vi "PathPlanner_Ctrl_HolonomicDrvExecute.vi"(6 "Period":dbl=0.02, 7 "PathPlanner_Ctrl_HolDrvConfig":T10={"HOLONOMIC_CTRL_PACK_TUNING"={"X PID Tuning"={"Kp"=0.0, "Ki"=0.0, "Kd"=0.0, "MaximumIntegral"=9.9e+30, "MinimumIntegral"=-9.9e+30}, "Y PID Tuning"={"Kp"=0.0, "Ki"=0.0, "Kd"=0.0, "MaximumIntegral"=9.9e+30, "MinimumIntegral"=-9.9e+30}, "thetaProfiledPID_CTRL"={"Controller"={"Kp"=0.0, "Ki"=0.0, "Kd"=0.0, "Period"=0.0, "Max_Integral"=1.0, "Min_Integral"=-1.0, "Max_Input"=0.0, "Min_Input"=0.0, "Continuous"=FALSE, "PositionError"=0.0, "VelocityError"=0.0, "PrevError"=0.0, "TotalError"=0.0, "PositionTolerance"=0.05, "VelocityTolerance"=9.99e+35, "SetPoint"=0.0, "Kf"=0.0, "Prev_Deriv"=0.0, "Prev_Deriv 2"=0.0, "DerivativeFilter"=FALSE, "Min_Output"=-9.99e+35, "Max_Output"=9.9e+35, "Prev_F_P"=0.0, "Prev_F_P_2"=0.0, "AntiWindupActive"=FALSE, "Measurement"=0.0}, "Goal"={"Position"=0.0, "Velocity"=0.0}, "Setpoint"={"Position"=0.0, "Velocity"=0.0}, "Constraint"={"MaxVelocity"=0.0, "MaxAcceleration"=0.0}}}, "Max Wheel Speed M/S"=0.0, "Tolerance SI"={"TRANSLATION"={"X"=0.04, "Y"=0.04}, "ROTATION"={"VALUE"=0.034906585039887, "COS"=0.999390827019096, "SIN"=0.034899496702501}}, "Drive Base Radius M"=0.0} {"Tolerance SI"."ROTATION"."SIN" format="%13.4f"; "Tolerance SI"."ROTATION"."COS" format="%13.4f"; "Tolerance SI"."ROTATION"."VALUE" format="%13.4f"; "Tolerance SI"."TRANSLATION"."Y" format="%14.3f"; "Tolerance SI"."TRANSLATION"."X" format="%14.3f"; "HOLONOMIC_CTRL_PACK_TUNING"."thetaProfiledPID_CTRL"."Constraint"."MaxAcceleration" format="%16_6e"; "HOLONOMIC_CTRL_PACK_TUNING"."thetaProfiledPID_CTRL"."Constraint"."MaxVelocity" format="%16_6e"; "HOLONOMIC_CTRL_PACK_TUNING"."thetaProfiledPID_CTRL"."Setpoint"."Velocity" format="%16_6e"; "HOLONOMIC_CTRL_PACK_TUNING"."thetaProfiledPID_CTRL"."Setpoint"."Position" format="%16_6e"; "HOLONOMIC_CTRL_PACK_TUNING"."thetaProfiledPID_CTRL"."Goal"."Velocity" format="%16_6e"; "HOLONOMIC_CTRL_PACK_TUNING"."thetaProfiledPID_CTRL"."Goal"."Position" format="%16_6e"; "HOLONOMIC_CTRL_PACK_TUNING"."thetaProfiledPID_CTRL"."Controller"."Measurement" format="%16_6e"; "HOLONOMIC_CTRL_PACK_TUNING"."thetaProfiledPID_CTRL"."Controller"."Prev_F_P_2" format="%16_6e"; "HOLONOMIC_CTRL_PACK_TUNING"."thetaProfiledPID_CTRL"."Controller"."Prev_F_P" format="%16_6e"; "HOLONOMIC_CTRL_PACK_TUNING"."thetaProfiledPID_CTRL"."Controller"."Max_Output" format="%16_6e"; "HOLONOMIC_CTRL_PACK_TUNING"."thetaProfiledPID_CTRL"."Controller"."Min_Output" format="%16_6e"; "HOLONOMIC_CTRL_PACK_TUNING"."thetaProfiledPID_CTRL"."Controller"."Prev_Deriv 2" format="%16_6e"; "HOLONOMIC_CTRL_PACK_TUNING"."thetaProfiledPID_CTRL"."Controller"."Prev_Deriv" format="%16_6e"; "HOLONOMIC_CTRL_PACK_TUNING"."thetaProfiledPID_CTRL"."Controller"."Kf" format="%16_6e"; "HOLONOMIC_CTRL_PACK_TUNING"."thetaProfiledPID_CTRL"."Controller"."SetPoint" format="%16_6e"; "HOLONOMIC_CTRL_PACK_TUNING"."thetaProfiledPID_CTRL"."Controller"."VelocityTolerance" format="%16_6e"; "HOLONOMIC_CTRL_PACK_TUNING"."thetaProfiledPID_CTRL"."Controller"."PositionTolerance" format="%16_6e"; "HOLONOMIC_CTRL_PACK_TUNING"."thetaProfiledPID_CTRL"."Controller"."TotalError" format="%16_6e"; "HOLONOMIC_CTRL_PACK_TUNING"."thetaProfiledPID_CTRL"."Controller"."PrevError" format="%16_6e"; "HOLONOMIC_CTRL_PACK_TUNING"."thetaProfiledPID_CTRL"."Controller"."VelocityError" format="%16_6e"; "HOLONOMIC_CTRL_PACK_TUNING"."thetaProfiledPID_CTRL"."Controller"."PositionError" format="%16_6e"; "HOLONOMIC_CTRL_PACK_TUNING"."thetaProfiledPID_CTRL"."Controller"."Min_Input" format="%16_6e"; "HOLONOMIC_CTRL_PACK_TUNING"."thetaProfiledPID_CTRL"."Controller"."Max_Input" format="%16_6e"; "HOLONOMIC_CTRL_PACK_TUNING"."thetaProfiledPID_CTRL"."Controller"."Min_Integral" format="%16_6e"; "HOLONOMIC_CTRL_PACK_TUNING"."thetaProfiledPID_CTRL"."Controller"."Max_Integral" format="%16_6e"; "HOLONOMIC_CTRL_PACK_TUNING"."thetaProfiledPID_CTRL"."Controller"."Period" format="%16_6e"; "HOLONOMIC_CTRL_PACK_TUNING"."thetaProfiledPID_CTRL"."Controller"."Kd" format="%16_6e"; "HOLONOMIC_CTRL_PACK_TUNING"."thetaProfiledPID_CTRL"."Controller"."Ki" format="%16_6e"; "HOLONOMIC_CTRL_PACK_TUNING"."thetaProfiledPID_CTRL"."Controller"."Kp" format="%16_6e"}, 8 "Enabled":bool=TRUE, 9 "Reset":bool, 10 "PathPlannerState":T13={"TimeSeconds"=0.0, "VelocityMPS"=0.0, "AccerationMpsSq"=0.0, "HeadingAngularVelRadPerSec"=0.0, "PositionMeters"={"X"=0.0, "Y"=0.0}, "Heading"={"VALUE"=0.0, "COS"=1.0, "SIN"=0.0}, "TargetHolonomicRotation"={"VALUE"=0.0, "COS"=1.0, "SIN"=0.0}, "CurvatureRadPerMeter"=0.0, "PathPlannerConstraints"={"MaxVelocityMps;"=0.0, "MaxAccelerationMpsSq;"=0.0, "MaxAngularVelRadPsEc;"=0.0, "MaxAngularAccRadPSecSq"=0.0, "Exists"=FALSE}, "DeltaPos"=0.0} {"TargetHolonomicRotation"."SIN" format="%13.4f"; "TargetHolonomicRotation"."COS" format="%13.4f"; "TargetHolonomicRotation"."VALUE" format="%13.4f"; "Heading"."SIN" format="%13.4f"; "Heading"."COS" format="%13.4f"; "Heading"."VALUE" format="%13.4f"; "PositionMeters"."Y" format="%14.3f"; "PositionMeters"."X" format="%14.3f"}, 11 "Current Pose SI":T3={"TRANSLATION"={"X"=0.0, "Y"=0.0}, "ROTATION"={"VALUE"=0.0, "COS"=1.0, "SIN"=0.0}} {"ROTATION"."SIN" format="%13.4f"; "ROTATION"."COS" format="%13.4f"; "ROTATION"."VALUE" format="%13.4f"; "TRANSLATION"."Y" format="%14.3f"; "TRANSLATION"."X" format="%14.3f"}) -> (1 "Position Error M":dbl, 2 "At Reference":bool, 3 "calcChassisSpeed":T1 {"vOmega" format="%10.3f"; "vY" format="%10.3f"; "vX" format="%10.3f"}, 4 "outHOLONOMIC_DRV_CTRL":T2={"poseTolerance"={"TRANSLATION"={"X"=0.0, "Y"=0.0}, "ROTATION"={"VALUE"=0.0, "COS"=1.0, "SIN"=0.0}}, "poseError"={"TRANSLATION"={"X"=0.0, "Y"=0.0}, "ROTATION"={"VALUE"=0.0, "COS"=1.0, "SIN"=0.0}}, "Enabled"=TRUE, "PID_xCtrl"={"Kp"=0.0, "Ki"=0.0, "Kd"=0.0, "Period"=0.0, "Max_Integral"=1.0, "Min_Integral"=-1.0, "Max_Input"=0.0, "Min_Input"=0.0, "Continuous"=FALSE, "PositionError"=0.0, "VelocityError"=0.0, "PrevError"=0.0, "TotalError"=0.0, "PositionTolerance"=0.05, "VelocityTolerance"=9.99e+35, "SetPoint"=0.0, "Kf"=0.0, "Prev_Deriv"=0.0, "Prev_Deriv 2"=0.0, "DerivativeFilter"=FALSE, "Min_Output"=-9.99e+35, "Max_Output"=9.9e+35, "Prev_F_P"=0.0, "Prev_F_P_2"=0.0, "AntiWindupActive"=FALSE, "Measurement"=0.0}, "PID_yCtrl"={"Kp"=0.0, "Ki"=0.0, "Kd"=0.0, "Period"=0.0, "Max_Integral"=1.0, "Min_Integral"=-1.0, "Max_Input"=0.0, "Min_Input"=0.0, "Continuous"=FALSE, "PositionError"=0.0, "VelocityError"=0.0, "PrevError"=0.0, "TotalError"=0.0, "PositionTolerance"=0.05, "VelocityTolerance"=9.99e+35, "SetPoint"=0.0, "Kf"=0.0, "Prev_Deriv"=0.0, "Prev_Deriv 2"=0.0, "DerivativeFilter"=FALSE, "Min_Output"=-9.99e+35, "Max_Output"=9.9e+35, "Prev_F_P"=0.0, "Prev_F_P_2"=0.0, "AntiWindupActive"=FALSE, "Measurement"=0.0}, "PROF_PID_thetaCtrl"={"Controller"={"Kp"=0.0, "Ki"=0.0, "Kd"=0.0, "Period"=0.0, "Max_Integral"=1.0, "Min_Integral"=-1.0, "Max_Input"=0.0, "Min_Input"=0.0, "Continuous"=FALSE, "PositionError"=0.0, "VelocityError"=0.0, "PrevError"=0.0, "TotalError"=0.0, "PositionTolerance"=0.05, "VelocityTolerance"=9.99e+35, "SetPoint"=0.0, "Kf"=0.0, "Prev_Deriv"=0.0, "Prev_Deriv 2"=0.0, "DerivativeFilter"=FALSE, "Min_Output"=-9.99e+35, "Max_Output"=9.9e+35, "Prev_F_P"=0.0, "Prev_F_P_2"=0.0, "AntiWindupActive"=FALSE, "Measurement"=0.0}, "Goal"={"Position"=0.0, "Velocity"=0.0}, "Setpoint"={"Position"=0.0, "Velocity"=0.0}, "Constraint"={"MaxVelocity"=0.0, "MaxAcceleration"=0.0}}, "RotationError"={"VALUE"=0.0, "COS"=1.0, "SIN"=0.0}, "FirstRun"=TRUE} {"RotationError"."SIN" format="%13.4f"; "RotationError"."COS" format="%13.4f"; "RotationError"."VALUE" format="%13.4f"; "PROF_PID_thetaCtrl"."Constraint"."MaxAcceleration" format="%16_6e"; "PROF_PID_thetaCtrl"."Constraint"."MaxVelocity" format="%16_6e"; "PROF_PID_thetaCtrl"."Setpoint"."Velocity" format="%16_6e"; "PROF_PID_thetaCtrl"."Setpoint"."Position" format="%16_6e"; "PROF_PID_thetaCtrl"."Goal"."Velocity" format="%16_6e"; "PROF_PID_thetaCtrl"."Goal"."Position" format="%16_6e"; "PROF_PID_thetaCtrl"."Controller"."Measurement" format="%16_6e"; "PROF_PID_thetaCtrl"."Controller"."Prev_F_P_2" format="%16_6e"; "PROF_PID_thetaCtrl"."Controller"."Prev_F_P" format="%16_6e"; "PROF_PID_thetaCtrl"."Controller"."Max_Output" format="%16_6e"; "PROF_PID_thetaCtrl"."Controller"."Min_Output" format="%16_6e"; "PROF_PID_thetaCtrl"."Controller"."Prev_Deriv 2" format="%16_6e"; "PROF_PID_thetaCtrl"."Controller"."Prev_Deriv" format="%16_6e"; "PROF_PID_thetaCtrl"."Controller"."Kf" format="%16_6e"; "PROF_PID_thetaCtrl"."Controller"."SetPoint" format="%16_6e"; "PROF_PID_thetaCtrl"."Controller"."VelocityTolerance" format="%16_6e"; "PROF_PID_thetaCtrl"."Controller"."PositionTolerance" format="%16_6e"; "PROF_PID_thetaCtrl"."Controller"."TotalError" format="%16_6e"; "PROF_PID_thetaCtrl"."Controller"."PrevError" format="%16_6e"; "PROF_PID_thetaCtrl"."Controller"."VelocityError" format="%16_6e"; "PROF_PID_thetaCtrl"."Controller"."PositionError" format="%16_6e"; "PROF_PID_thetaCtrl"."Controller"."Min_Input" format="%16_6e"; "PROF_PID_thetaCtrl"."Controller"."Max_Input" format="%16_6e"; "PROF_PID_thetaCtrl"."Controller"."Min_Integral" format="%16_6e"; "PROF_PID_thetaCtrl"."Controller"."Max_Integral" format="%16_6e"; "PROF_PID_thetaCtrl"."Controller"."Period" format="%16_6e"; "PROF_PID_thetaCtrl"."Controller"."Kd" format="%16_6e"; "PROF_PID_thetaCtrl"."Controller"."Ki" format="%16_6e"; "PROF_PID_thetaCtrl"."Controller"."Kp" format="%16_6e"; "PID_yCtrl"."Measurement" format="%16_6e"; "PID_yCtrl"."Prev_F_P_2" format="%16_6e"; "PID_yCtrl"."Prev_F_P" format="%16_6e"; "PID_yCtrl"."Max_Output" format="%16_6e"; "PID_yCtrl"."Min_Output" format="%16_6e"; "PID_yCtrl"."Prev_Deriv 2" format="%16_6e"; "PID_yCtrl"."Prev_Deriv" format="%16_6e"; "PID_yCtrl"."Kf" format="%16_6e"; "PID_yCtrl"."SetPoint" format="%16_6e"; "PID_yCtrl"."VelocityTolerance" format="%16_6e"; "PID_yCtrl"."PositionTolerance" format="%16_6e"; "PID_yCtrl"."TotalError" format="%16_6e"; "PID_yCtrl"."PrevError" format="%16_6e"; "PID_yCtrl"."VelocityError" format="%16_6e"; "PID_yCtrl"."PositionError" format="%16_6e"; "PID_yCtrl"."Min_Input" format="%16_6e"; "PID_yCtrl"."Max_Input" format="%16_6e"; "PID_yCtrl"."Min_Integral" format="%16_6e"; "PID_yCtrl"."Max_Integral" format="%16_6e"; "PID_yCtrl"."Period" format="%16_6e"; "PID_yCtrl"."Kd" format="%16_6e"; "PID_yCtrl"."Ki" format="%16_6e"; "PID_yCtrl"."Kp" format="%16_6e"; "PID_xCtrl"."Measurement" format="%16_6e"; "PID_xCtrl"."Prev_F_P_2" format="%16_6e"; "PID_xCtrl"."Prev_F_P" format="%16_6e"; "PID_xCtrl"."Max_Output" format="%16_6e"; "PID_xCtrl"."Min_Output" format="%16_6e"; "PID_xCtrl"."Prev_Deriv 2" format="%16_6e"; "PID_xCtrl"."Prev_Deriv" format="%16_6e"; "PID_xCtrl"."Kf" format="%16_6e"; "PID_xCtrl"."SetPoint" format="%16_6e"; "PID_xCtrl"."VelocityTolerance" format="%16_6e"; "PID_xCtrl"."PositionTolerance" format="%16_6e"; "PID_xCtrl"."TotalError" format="%16_6e"; "PID_xCtrl"."PrevError" format="%16_6e"; "PID_xCtrl"."VelocityError" format="%16_6e"; "PID_xCtrl"."PositionError" format="%16_6e"; "PID_xCtrl"."Min_Input" format="%16_6e"; "PID_xCtrl"."Max_Input" format="%16_6e"; "PID_xCtrl"."Min_Integral" format="%16_6e"; "PID_xCtrl"."Max_Integral" format="%16_6e"; "PID_xCtrl"."Period" format="%16_6e"; "PID_xCtrl"."Kd" format="%16_6e"; "PID_xCtrl"."Ki" format="%16_6e"; "PID_xCtrl"."Kp" format="%16_6e"; "poseError"."ROTATION"."SIN" format="%13.4f"; "poseError"."ROTATION"."COS" format="%13.4f"; "poseError"."ROTATION"."VALUE" format="%13.4f"; "poseError"."TRANSLATION"."Y" format="%14.3f"; "poseError"."TRANSLATION"."X" format="%14.3f"; "poseTolerance"."ROTATION"."SIN" format="%13.4f"; "poseTolerance"."ROTATION"."COS" format="%13.4f"; "poseTolerance"."ROTATION"."VALUE" format="%13.4f"; "poseTolerance"."TRANSLATION"."Y" format="%14.3f"; "poseTolerance"."TRANSLATION"."X" format="%14.3f"})   [LabVIEW 2019]
doc: "Calculates the next output of the path following controller for holonomic drive robots. This wraps a Holonomic Drive Control function with the particulars needed to follow a PathPlanner trajectory.\n\nInputs:\n - PathPlanner_Holonomic_Ctrl_Pack_Tuning - cluster - The tuning paraameters for the holonomic drive controller. These are static. They should not be changed after the first call to this function.\n - CurrentPoseSi - pose2d - The current pose calculated by odometry or pose estimation. The pose can be absolute or relative depending on what type of trajectory is being followed.\n - PathPlannerState - cluster - The path palnner trajectory state containing the desired position and velocities of the robot.\n - Reset - boolean - When TRUE the holonomic drive controller is reset. This should be set to TRUE for the first execution of a trajectory.\n - Enabled - boolean - When TRUE, closed loop control is enabled. (Optional. Default: TRUE)\n - Period - double - The loop period in seconds for this controller. (Optional. Default: 0.020)\n\nOutputs:\n - CalcChassisSpeed - cluster - The desired chassis speed in SI units.\n - AtReference - boolean - TRUE if the robots position is within the defined tolerance.\n - PositionError - pose2d - Position error in SI units. How far the robot is away from the desired trajectory position.\n - out_Holonomic_Drive_Ctrl - THe current holonomic drive controller data cluster. This is mainly for diagnostic purposes."
uses:
  <vilib>/Rock Robotics/WPI/ThirdParty/JAS_Junk/TrajLib/Trajectory_Library.lvlib
  <vilib>/Rock Robotics/WPI/ThirdParty/JAS_Junk/TrajLib/TypeDef/TRANSLATION2D.ctl
  <vilib>/Rock Robotics/WPI/ThirdParty/JAS_Junk/TrajLib/TypeDef/ROTATION2D.ctl
  <vilib>/Rock Robotics/WPI/ThirdParty/JAS_Junk/TrajLib/TypeDef/POSE2D.ctl
  TypeDef/PathPlannerPathConstraints.ctl
  TypeDef/PathPlannerTrajectoryState.ctl
  <vilib>/Rock Robotics/WPI/ThirdParty/JAS_Junk/TrajLib/TypeDef/PID_TUNING.ctl
  <vilib>/Rock Robotics/WPI/ThirdParty/JAS_Junk/TrajLib/TypeDef/PID_CONTROLLER.ctl
  <vilib>/Rock Robotics/WPI/ThirdParty/JAS_Junk/TrajLib/TypeDef/TRAPEZOID_PROFILE_STATE.ctl
  <vilib>/Rock Robotics/WPI/ThirdParty/JAS_Junk/TrajLib/TypeDef/TRAPEZOID_PROFILE_CONSTRAINT.ctl
  <vilib>/Rock Robotics/WPI/ThirdParty/JAS_Junk/TrajLib/TypeDef/PROFILED_PID_CONTROLLER.ctl
  <vilib>/Rock Robotics/WPI/ThirdParty/JAS_Junk/TrajLib/TypeDef/HOLONOMIC_PACK_TUNING.ctl
  <vilib>/Rock Robotics/WPI/ThirdParty/JAS_Junk/TrajLib/TypeDef/HOLONOMIC_DRV_CTRL.ctl
  <vilib>/Rock Robotics/WPI/ThirdParty/JAS_Junk/TrajLib/TypeDef/CHASSIS_SPEEDS.ctl
  TypeDef/PathPlannerCtrlHolConfig.ctl
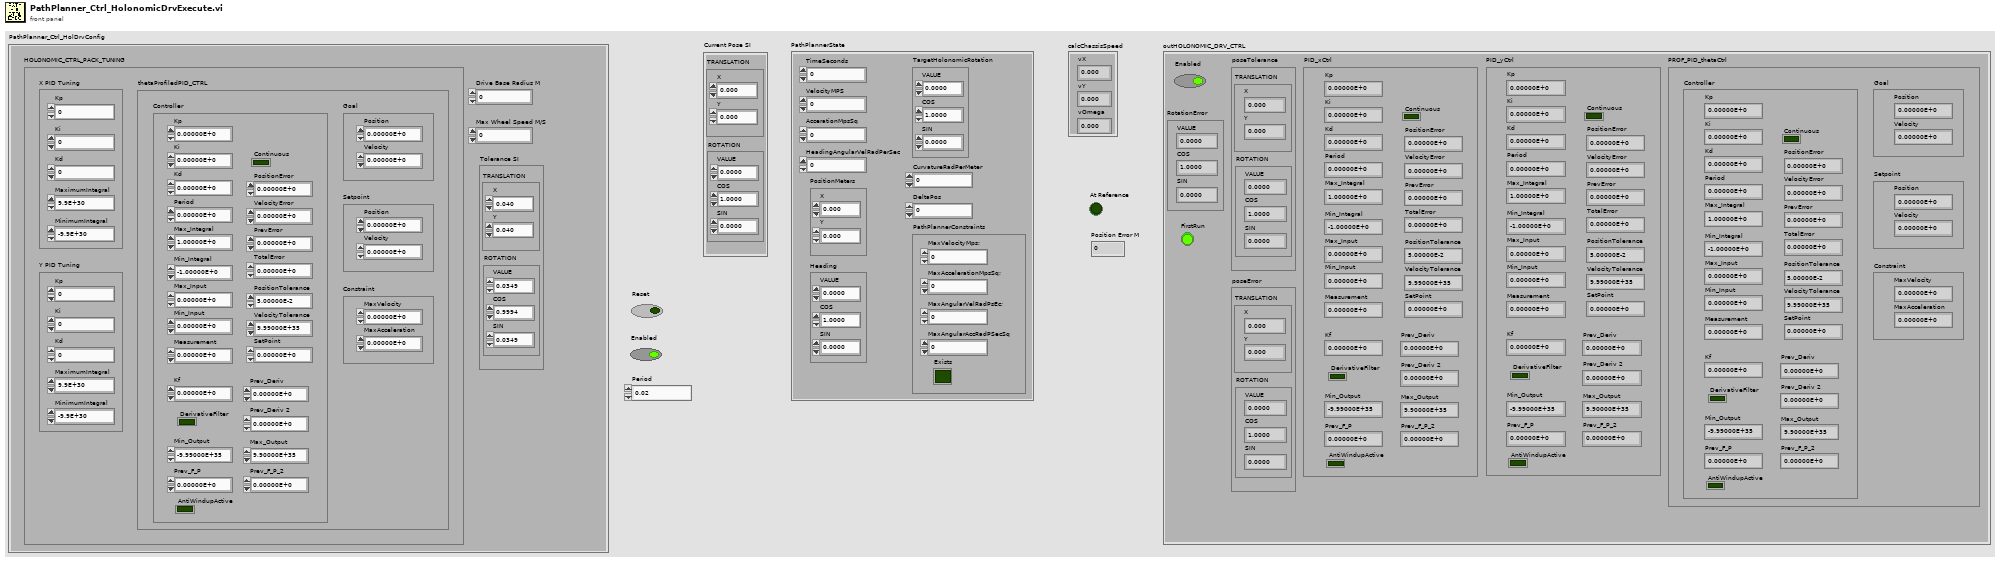
[diagram p1: front panel]
types:
  T1 = typedef "Trajectory_Library.lvlib/CHASSIS_SPEEDS.ctl" = cluster{"vX":dbl, "vY":dbl, "vOmega":dbl}
  T2 = typedef "Trajectory_Library.lvlib/HOLONOMIC_DRV_CTRL.ctl" = cluster{"poseTolerance":T3, "poseError":T3, "Enabled":bool, "PID_xCtrl":T6, "PID_yCtrl":T6, "PROF_PID_thetaCtrl":T7, "RotationError":T5, "FirstRun":bool}
  T3 = typedef "Trajectory_Library.lvlib/POSE2D.ctl" = cluster{"TRANSLATION":T4, "ROTATION":T5}
  T4 = typedef "Trajectory_Library.lvlib/TRANSLATION2D.ctl" = cluster{"X":dbl, "Y":dbl}
  T5 = typedef "Trajectory_Library.lvlib/ROTATION2D.ctl" = cluster{"VALUE":dbl, "COS":dbl, "SIN":dbl}
  T6 = typedef "Trajectory_Library.lvlib/PID_CONTROLLER.ctl" = cluster{"Kp":dbl, "Ki":dbl, "Kd":dbl, "Period":dbl, "Max_Integral":dbl, "Min_Integral":dbl, "Max_Input":dbl, "Min_Input":dbl, "Continuous":bool, "PositionError":dbl, "VelocityError":dbl, "PrevError":dbl, "TotalError":dbl, "PositionTolerance":dbl, "VelocityTolerance":dbl, "SetPoint":dbl, "Kf":dbl, "Prev_Deriv":dbl, "Prev_Deriv 2":dbl, "DerivativeFilter":bool, "Min_Output":dbl, "Max_Output":dbl, "Prev_F_P":dbl, "Prev_F_P_2":dbl, "AntiWindupActive":bool, "Measurement":dbl}
  T7 = typedef "Trajectory_Library.lvlib/PROFILED_PID_CONTROLLER.ctl" = cluster{"Controller":T6, "Goal":T8, "Setpoint":T8, "Constraint":T9}
  T8 = typedef "Trajectory_Library.lvlib/TRAPEZOID_PROFILE_STATE.ctl" = cluster{"Position":dbl, "Velocity":dbl}
  T9 = typedef "Trajectory_Library.lvlib/TRAPEZOID_PROFILE_CONSTRAINT.ctl" = cluster{"MaxVelocity":dbl, "MaxAcceleration":dbl}
  T10 = typedef "PathPlannerCtrlHolConfig.ctl" = cluster{"HOLONOMIC_CTRL_PACK_TUNING":T11, "Max Wheel Speed M/S":dbl, "Tolerance SI":T3, "Drive Base Radius M":dbl}
  T11 = typedef "Trajectory_Library.lvlib/HOLONOMIC_PACK_TUNING.ctl" = cluster{"X PID Tuning":T12, "Y PID Tuning":T12, "thetaProfiledPID_CTRL":T7}
  T12 = typedef "Trajectory_Library.lvlib/PID_TUNING.ctl" = cluster{"Kp":dbl, "Ki":dbl, "Kd":dbl, "MaximumIntegral":dbl, "MinimumIntegral":dbl}
  T13 = typedef "PathPlannerTrajectoryState.ctl" = cluster{"TimeSeconds":dbl, "VelocityMPS":dbl, "AccerationMpsSq":dbl, "HeadingAngularVelRadPerSec":dbl, "PositionMeters":T4, "Heading":T5, "TargetHolonomicRotation":T5, "CurvatureRadPerMeter":dbl, "PathPlannerConstraints":T14, "DeltaPos":dbl}
  T14 = typedef "PathPlannerPathConstraints.ctl" = cluster{"MaxVelocityMps;":dbl, "MaxAccelerationMpsSq;":dbl, "MaxAngularVelRadPsEc;":dbl, "MaxAngularAccRadPSecSq":dbl, "Exists":bool}
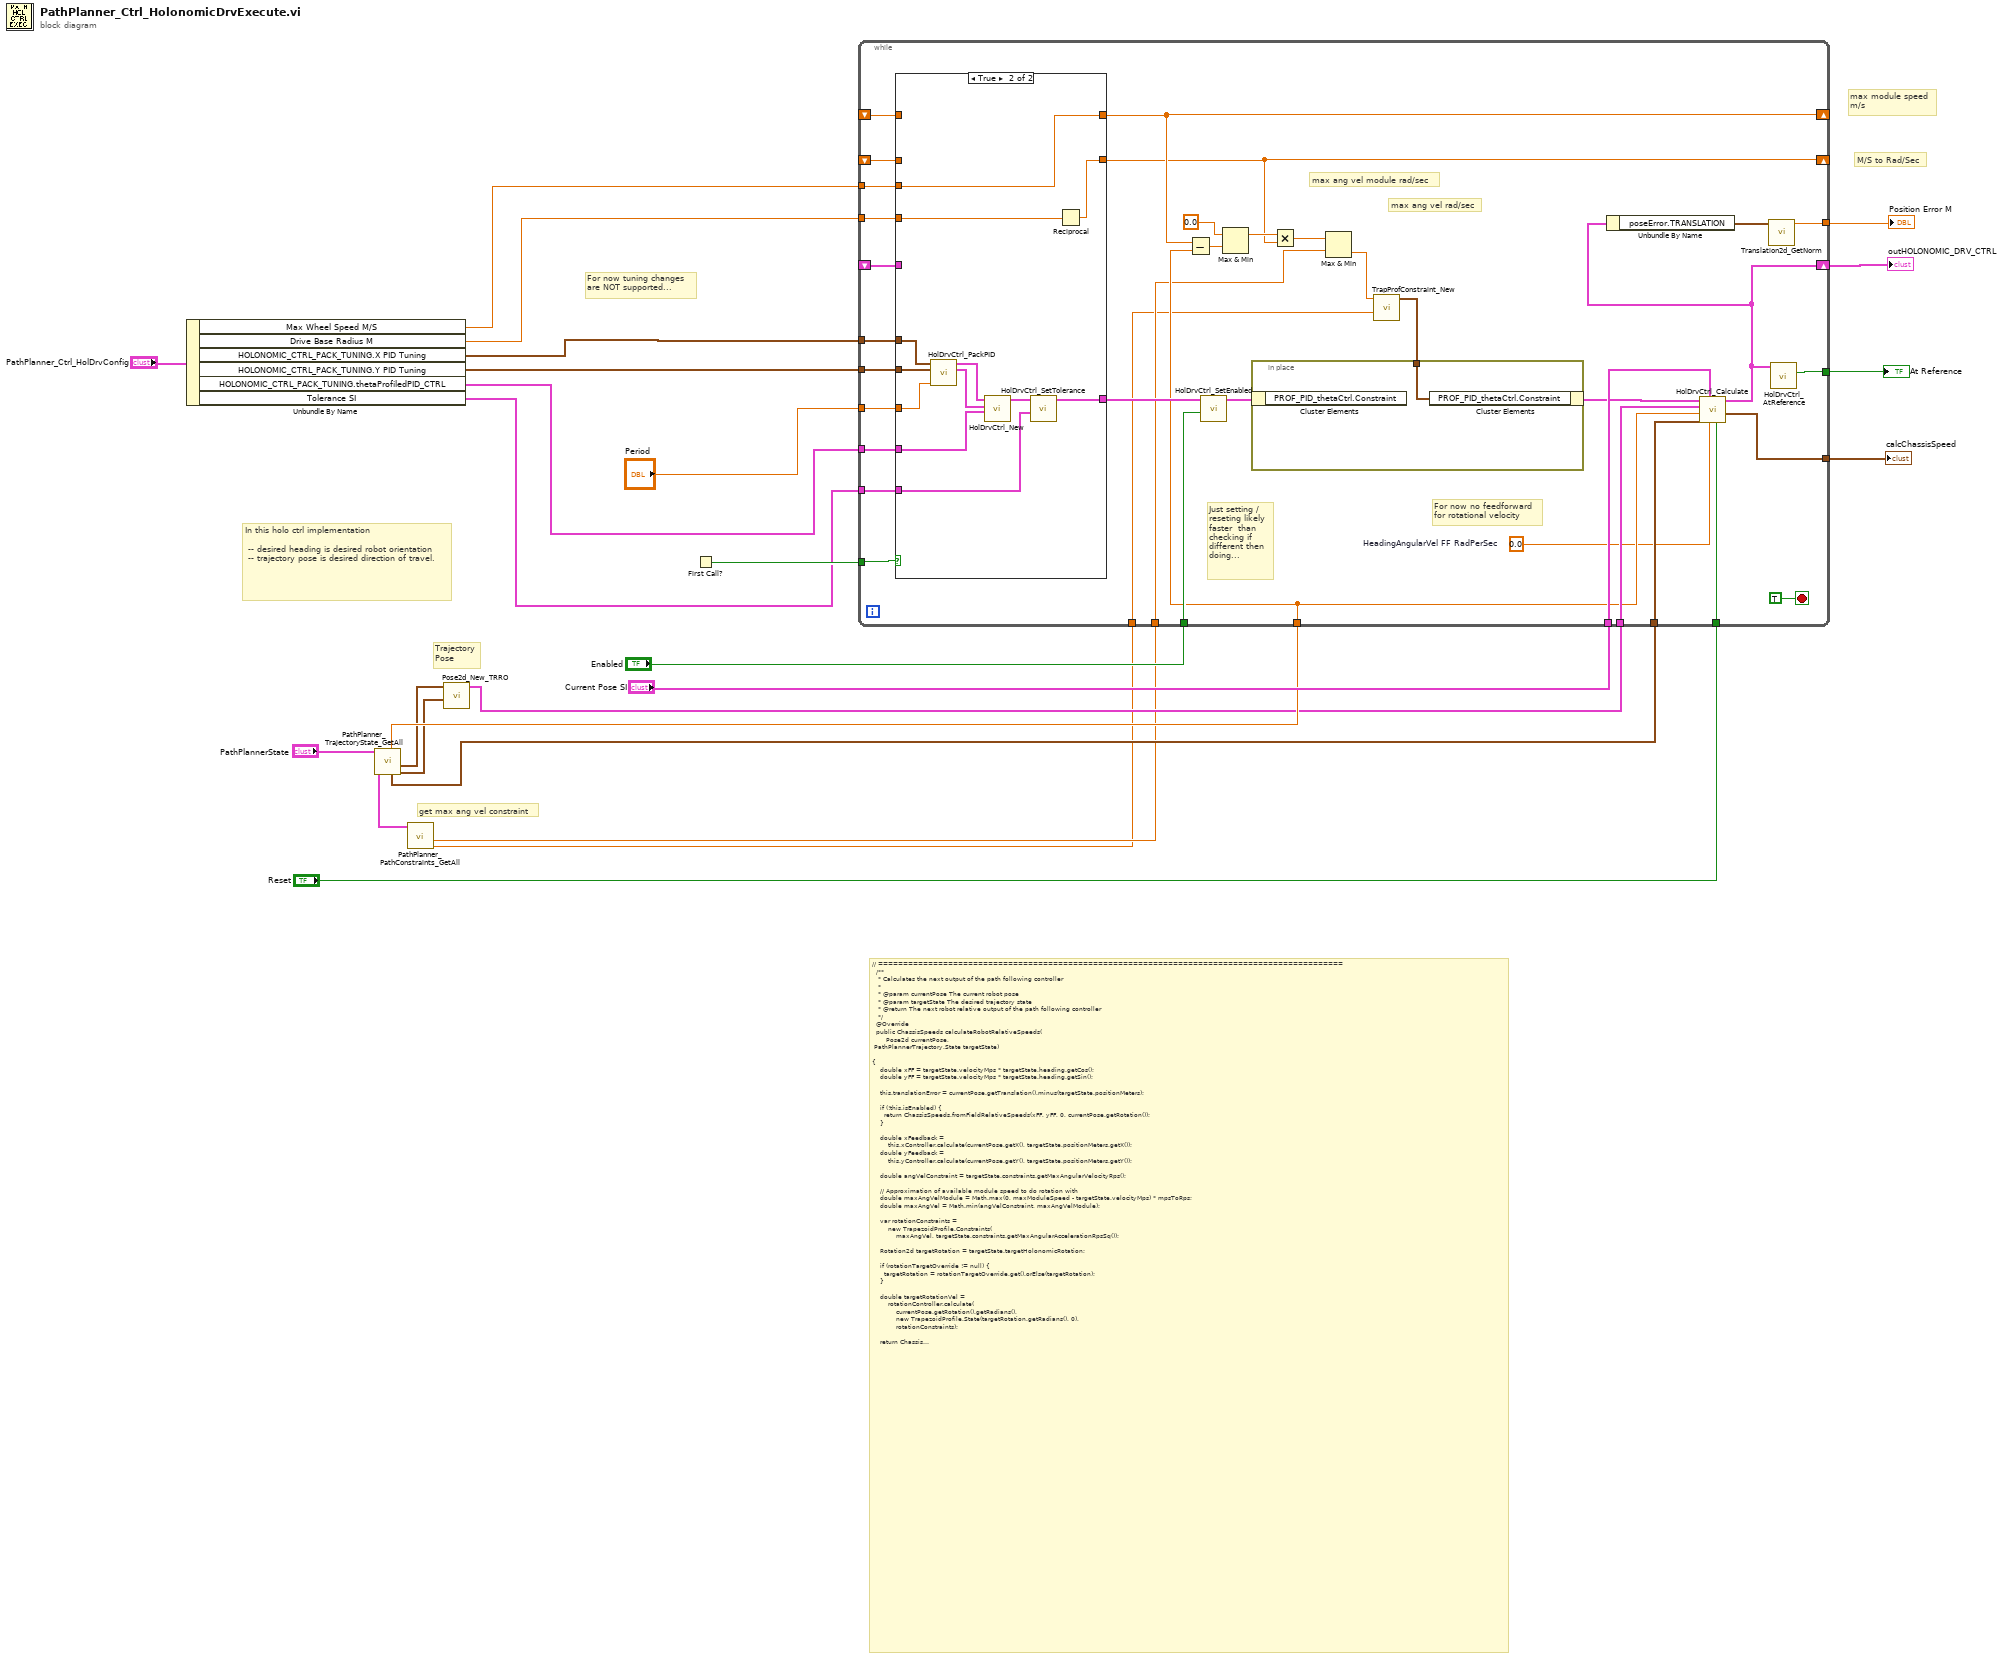
[diagram p0: block diagram]
diagram:
  # "get max ang vel constraint"
  # "M/S to Rad/Sec"
  # "max module speed\nm/s"
  # "Trajectory\nPose"
  # "// =============================================================================================\n  /**\n   * Calculates the next output of the path following controller\n   *\n   * @param currentPose The current robot pose\n   * @param targetState The desired trajectory state\n   * @return The next robot relative output of the path following controller\n   */\n  @Override\n  public ChassisSpeeds calculateRobotRelativeSpeeds(\n      \tPose2d currentPose, \n\tPathPlannerTrajectory.State targetState) \n\n{\n    double xFF = targetState.velocityMps * targetState.heading.getCos();\n    double yFF = targetState.velocityMps * targetState.heading.getSin();\n\n    this.translationError = currentPose.getTranslation().minus(targetState.positionMeters);\n\n    if (!this.isEnabled) {\n      return ChassisSpeeds.fromFieldRelativeSpeeds(xFF, yFF, 0, currentPose.getRotation());\n    }\n\n    double xFeedback =\n        this.xController.calculate(currentPose.getX(), targetState.positionMeters.getX());\n    double yFeedback =\n        this.yController.calculate(currentPose.getY(), targetState.positionMeters.getY());\n\n    double angVelConstraint = targetState.constraints.getMaxAngularVelocityRps();\n\n    // Approximation of available module speed to do rotation with\n    double maxAngVelModule = Math.max(0, maxModuleSpeed - targetState.velocityMps) * mpsToRps;\n    double maxAngVel = Math.min(angVelConstraint, maxAngVelModule);\n\n    var rotationConstraints =\n        new TrapezoidProfile.Constraints(\n            maxAngVel, targetState.constraints.getMaxAngularAccelerationRpsSq());\n\n    Rotation2d targetRotation = targetState.targetHolonomicRotation;\n\n    if (rotationTargetOverride != null) {\n      targetRotation = rotationTargetOverride.get().orElse(targetRotation);\n    }\n\n    double targetRotationVel =\n        rotationController.calculate(\n            currentPose.getRotation().getRadians(),\n            new TrapezoidProfile.State(targetRotation.getRadians(), 0),\n            rotationConstraints);\n\n    return ChassisSpeeds.fromFieldRelativeSpeeds(\n        xFF + xFeedback, \n        yFF + yFeedback, \n        targetRotationVel, currentPose.getRotation());\n  }"
  # "In this holo ctrl implementation\n\n -- desired heading is desired robot orientation\n -- trajectory pose is desired direction of travel."
  # "For now tuning changes\nare NOT supported..."
  n1 = Unbundle By Name("PathPlanner_Ctrl_HolDrvConfig") -> ("Max Wheel Speed M/S"=w3:dbl, "Drive Base Radius M"=w2:dbl, "HOLONOMIC_CTRL_PACK_TUNING.X PID Tuning"=w23:T12, "HOLONOMIC_CTRL_PACK_TUNING.Y PID Tuning"=w22:T12, "HOLONOMIC_CTRL_PACK_TUNING.thetaProfiledPID_CTRL"=w21:T7, "Tolerance SI"=w1:T3)
  n2 = call "PathPlanner_TrajectoryState_GetAll.vi"("PathPlannerState"="PathPlannerState") -> ("Heading"=w9:T5, "PositionMeters"=w10:T4, "TargetHolonomicRotation"=w7:T5, "VelocityMPS"=w11:dbl, "PathPlannerConstraints"=w6:T14)  [unwired: 1 in, 5 out]
  n3 = call "PathPlanner_PathConstraints_GetAll.vi"("PathPlannerConstraints"=w6) -> ("MaxAngularAccRadPSecSq"=w4:dbl, "MaxAngularVelRadPsEc;"=w5:dbl)  [unwired: 6 in, 3 out]
  n4 = call <vilib>:"Pose2d_New_TRRO.vi"("ROTATION"=w9, "TRANSLATION"=w10) -> ("outPOSE"=w8:T3)  [unwired: 9 in]
  n5 = First Call?() -> (First Call?: T/F=w25:bool)
  n6 = while {
    tunnel: w25 -> [w62]
    tunnel: w21 -> [w61]
    tunnel: "Enabled" -> [w59]
    tunnel: "Current Pose SI" -> [w51]
    tunnel: [w49] -> w14
    tunnel: w23 -> [w58]
    tunnel: w22 -> [w57]
    tunnel: "Period" -> [w56]
    shift-right: [w48] -> w15
    shift-left: _ -> [w54]
    tunnel: [w53] -> w16
    tunnel: w1 -> [w52]
    tunnel: "Reset" -> [w50]
    tunnel: [w46] -> w13
    tunnel: w8 -> [w45]
    tunnel: w11 -> [w40]
    tunnel: w7 -> [w44]
    shift-right: [w41] -> _
    shift-left: _ -> [w43]
    shift-right: [w36] -> _
    shift-left: _ -> [w42]
    tunnel: w5 -> [w34]
    tunnel: w4 -> [w29]
    tunnel: w3 -> [w27]
    tunnel: w2 -> [w26]
    stop <- TRUE stop-if-true
    w28 = 0.0  # HeadingAngularVel FF RadPerSec
    # "For now no feedforward\nfor rotational velocity"
    # "max ang vel rad/sec"
    # "max ang vel module rad/sec"
    # "Just setting /\nreseting likely \nfaster  than \nchecking if \ndifferent then \ndoing..."
    n7 = case shown="True" w62 {
      tunnel: w61 -> [_ w78]
      tunnel: [w66 w70] -> w60
      tunnel: w58 -> [_ w75]
      tunnel: w57 -> [_ w74]
      tunnel: w56 -> [_ w73]
      tunnel: w54 -> [w66 _]
      tunnel: w52 -> [_ w72]
      tunnel: [w65 w68] -> w41
      tunnel: w43 -> [w65 _]
      tunnel: [w64 w69] -> w36
      tunnel: w42 -> [w64 _]
      tunnel: w27 -> [_ w68]
      tunnel: w26 -> [_ w67]
      frame False {
        # "#TODO Check for tuning\nchanges and update..."
      }
      frame True {
        n8 = call <vilib>:"HolDrvCtrl_PackPID.vi"("Period"=w73, "Y PID Tuning"=w74, "X PID Tuning"=w75) -> ("Y PID CONTROLLER"=w76:T6, "X PID_CONTROLLER"=w77:T6)  [unwired: 7 in]
        n9 = call <vilib>:"HolDrvCtrl_New.vi"("thetaProfiledPID_CTRL"=w78, "yPID_CTRL"=w76, "xPID_CTRL"=w77) -> ("outHOLONOMIC_DRV_CTRL"=w71:T2)  [unwired: 8 in]
        n10 = call <vilib>:"HolDrvCtrl_SetTolerance.vi"("poseTolerance"=w72, "inHOLONOMIC_DRV_CTRL"=w71) -> ("outHOLONOMIC_DRV_CTRL"=w70:T2)  [unwired: 9 in]
        n11 = Reciprocal(x=w67) -> (1/x=w69:dbl)
      }
    }
    n12 = Subtract(x=w41, y=w40) -> (x-y=w39:dbl)
    n13 = call <vilib>:"HolDrvCtrl_SetEnabled.vi"("Enabled"=w59, "inHOLONOMIC_DRV_CTRL"=w60) -> ("outHOLONOMIC_DRV_CTRL"=w33:T2)  [unwired: 9 in]
    n14 = Max & Min(x=0.0, y=w39) -> (max(x,y)=w37:dbl)  [unwired: 1 out]
    n15 = Multiply(x=w37, y=w36) -> (x*y=w35:dbl)
    n16 = Max & Min(x=w35, y=w34) -> (min(x,y)=w30:dbl)  [unwired: 1 out]
    n17 = call <vilib>:"TrapProfConstraint_New.vi"("Max Accel"=w29, "Max Speed (M/S)"=w30) -> ("TRAPEZOID_PROFILE_CONSTRAINT"=w31:T9)  [unwired: 9 in]
    n18 = in-place {
      in-place-border: w31 -> [w63]
      n19 = in-place-cluster #1(w33) -> ()  [unwired: 1 out]
      n20 = in-place-cluster #1("PROF_PID_thetaCtrl.Constraint"=w63) -> (w32:T2)
    }
    n21 = call <vilib>:"HolDrvCtrl_Calculate.vi"("Reset"=w50, "Rotational Vel\nFF Rad/Sec"=w28, "currentPose"=w51, "desiredHeading"=w44, "desiredLinearVelocity\nMetersPerSecond"=w40, "trajectoryPose"=w45, "inHOLONOMIC_DRV_CTRL"=w32) -> ("calcChassisSpeed"=w49:T1, "outHOLONOMIC_DRV_CTRL"=w48:T2)  [unwired: 3 in]
    n22 = Unbundle By Name(w48) -> ("poseError.TRANSLATION"=w47:T4)
    n23 = call <vilib>:"Translation2d_GetNorm.vi"("In Translation"=w47) -> ("Norm"=w46:dbl)  [unwired: 10 in]
    n24 = call <vilib>:"HolDrvCtrl_AtReference.vi"("HOLONOMIC_DRV_CTRL"=w48) -> ("AtReference"=w53:bool)  [unwired: 10 in]
  }
  "At Reference" <- w16
  "Position Error M" <- w13
  "outHOLONOMIC_DRV_CTRL" <- w15
  "calcChassisSpeed" <- w14
